vi "String To String (RAW).vi"(8 "error in (no error)":errorcluster, 10 "String":string, 11 "Registry Object":refnum<class "Carya Config.lvclass">) -> (0 "error out":errorcluster, 2 "String (RAW)":string, 3 "Registry Object":refnum<class "Carya Config.lvclass">)   [LabVIEW 2013, in "Carya Config.lvclass"]
doc: "Copyright 2018, Carya Automatisering, Wiebe Walstra."
uses:
  Carya Config.lvclass
  <vilib>/regexp/Match Regular Expression.xnode
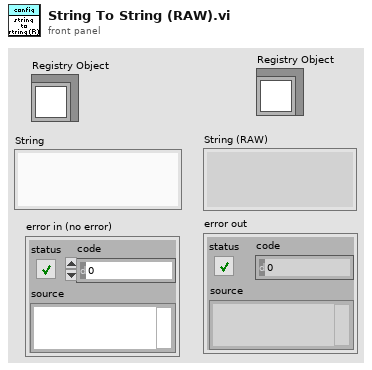
[diagram p1: front panel]
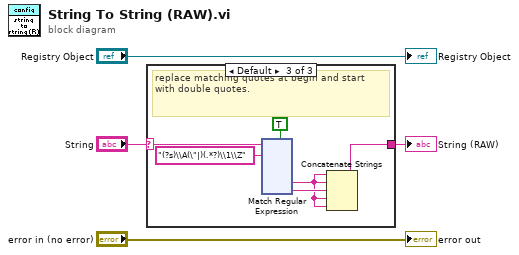
[diagram p0: block diagram]
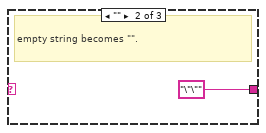
[diagram p3: hidden frame]
diagram:
  n1 = case shown="Default" "String" {
    selector: "String" -> [w5 _ w11]
    tunnel: [w5 "\"\"" ("result string") w9] -> w2
    frame "\"" {
      # "\" stays \"."
    }
    frame "" {
      # "empty string becomes \"\"."
    }
    frame Default {
      # "replace matching quotes at begin and start with double quotes."
      n2 = xnode "Match Regular Expression"("input string"=w11, "regular expression"="(?s)\\A(\"|)(.*?)\\1\\Z", "multiline? (F)"=TRUE) -> ("submatch 1"=w8:string, "submatch 2"=w10:string)  [unwired: 3 in, 5 out]
      n3 = Concatenate Strings(w8, w8, w10, w8, w8) -> (w9:string)
    }
  }
  "String (RAW)" <- w2
  "Registry Object" <- "Registry Object"
  "error out" <- "error in (no error)"
